vi "Vision Processing.vi"(4 "error in (no error)":errorcluster, 7 "Image Size":T6=enum."320x240") -> ()   [LabVIEW 2015]
doc: "This VI runs in parallel to other tasks. It gets images from the camera, processes them for color or shape and use that information to affect robot behavior."
uses:
  <vilib>/Rock Robotics/WPI/Camera/WPI_CameraImageSize.ctl
  Vision Example/Vision Support Code/Camera Types.ctl
  <vilib>/Rock Robotics/WPI/Camera/WPI_CameraWhite Balance Values.ctl
  <vilib>/Rock Robotics/WPI/Camera/WPI_CameraExposure Values.ctl
  <vilib>/Rock Robotics/WPI/Camera/WPI_CameraFrameRate.ctl
  Robot Global Data.vi
  <vilib>/vision/NI_Vision_Development_Module.lvlib
panel:
  out "ms to process":u32
  in  "LED Color":T1={"Hue"={23.67058792990901, 48.923317529462665}, "Sat"={66.78571428571429, 255.0}, "Val"={48.571428571428584, 255.0}} {"Hue" scale=0.0..255.0 scale format="%#_3g"}
  out "Qualified Particles":i32
  in  "Score Threshold":dbl=75.0
  in  "Aspect Fudge Factor":dbl=1.0
  in  "Min Score Threshold":i32=75
  in  "Camera Type":T2=enum."MS HD3000 square"
  in  "Emphasize Limit Tests":bool=TRUE
  out "Masked":T3(plugin-control)
  in  "Display Mask":bool=TRUE
  out "Original Image":T3(plugin-control)
  in  "Display Original":bool=TRUE
  out "Sorted Particle Scores":T4(array[cluster]) {"Moment Factor" format="%#_3g"; "Aspect Ratio" format="%#_3g"; "Area to CH" format="%#_3g"; "X" format="%#_3g"; "Y" format="%#_3g"}
  out "Highest Avg Score":dbl
  out "Detected Targets":T5(array[cluster]) {"Normalized Rect"."Numeric 5" format="%#_2g"; "Normalized Rect"."Numeric 3" format="%#_2g"; "Normalized Rect"."Numeric 2" format="%#_2g"; "Normalized Rect"."Numeric" format="%#_2g"}
  out "fps":dbl
  # "Density Profile"
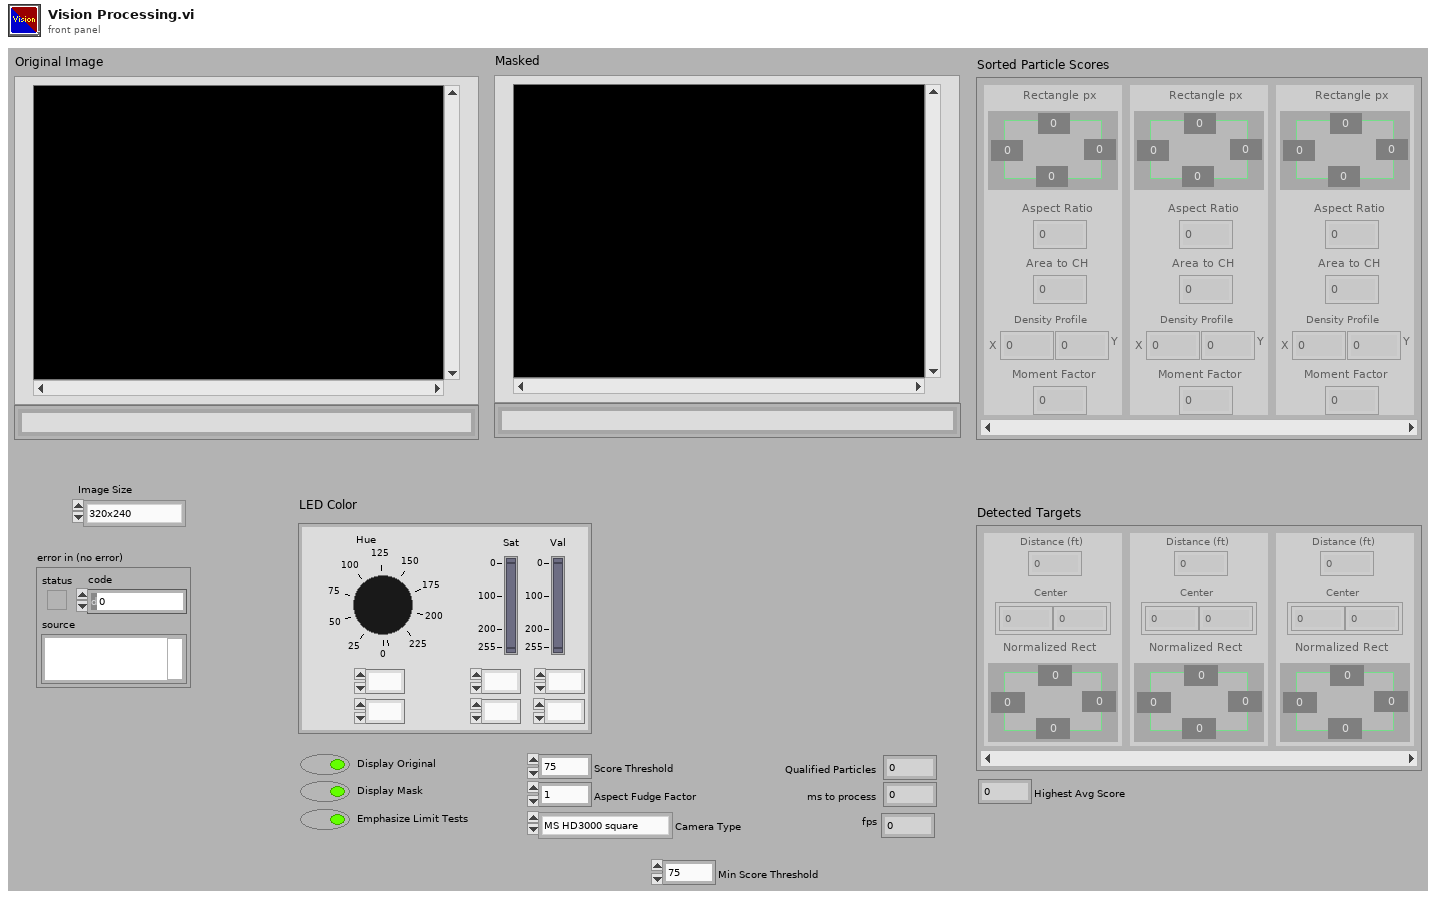
[diagram p1: front panel]
types:
  T1 = cluster{"Hue":cluster{dbl, dbl}, "Sat":cluster{dbl, dbl}, "Val":cluster{dbl, dbl}}
  T2 = typedef "Camera Types.ctl" = enum16{"206", "1011", "1013", "MS HD3000 square", "MS HD3000 640x480"}
  T3 = typedef "IMAQ Image.ctl" = refnum<image>
  T4 = cluster{"Rectangle px":cluster{"Numeric":dbl, "Numeric 2":dbl, "Numeric 3":dbl, "Numeric 5":dbl}, "Aspect Ratio":dbl, "Area to CH":dbl, "X":dbl, "Y":dbl, "Moment Factor":dbl}[]
  T5 = cluster{"Distance (ft)":dbl, "Center":cluster{dbl, dbl}, "Normalized Rect":cluster{"Numeric":dbl, "Numeric 2":dbl, "Numeric 3":dbl, "Numeric 5":dbl}}[]
  T6 = typedef "WPI_CameraImageSize.ctl" = enum16{"640x480", "320x240", "160x120", "Custom"}
  T7 = typedef "WPI_CameraFrameRate.ctl" = u32
  T8 = typedef "WPI_CameraExposure Values.ctl" = enum16{"Auto", "Flicker-free 50 Hz", "Flicker-free 60 Hz", "Hold current", "Custom"}
  T9 = typedef "WPI_CameraWhite Balance Values.ctl" = enum16{"Auto", "Fixed indoor", "Fixed outdoor 1", "Fixed outdoor 2", "Fixed fluorescent 1", "Fixed fluorescent 2", "Hold current", "Custom"}
  T10 = typedef "Particle Parameters" = i32
  T11 = typedef "Image Type" = u32
  T12 = typedef "WPI_CameraDevRef.ctl" = cluster{"Camera Address":string, "CameraStatus":errorcluster}
  T13 = cluster{"Bounding box":cluster{"left":dbl, "top":dbl, "right":dbl, "bottom":dbl}, "Aspect Ratio":dbl, "Area to CH":dbl, "X Mask":dbl, "Y Mask":dbl, "Moment":dbl}[]
  T14 = cluster{"Rectangle":cluster{"Numeric":dbl, "Numeric 2":dbl, "Numeric 3":dbl, "Numeric 5":dbl}, "L":dbl, "Area to CH":dbl, "X":dbl, "Y":dbl, "Moment Factor":dbl}[]
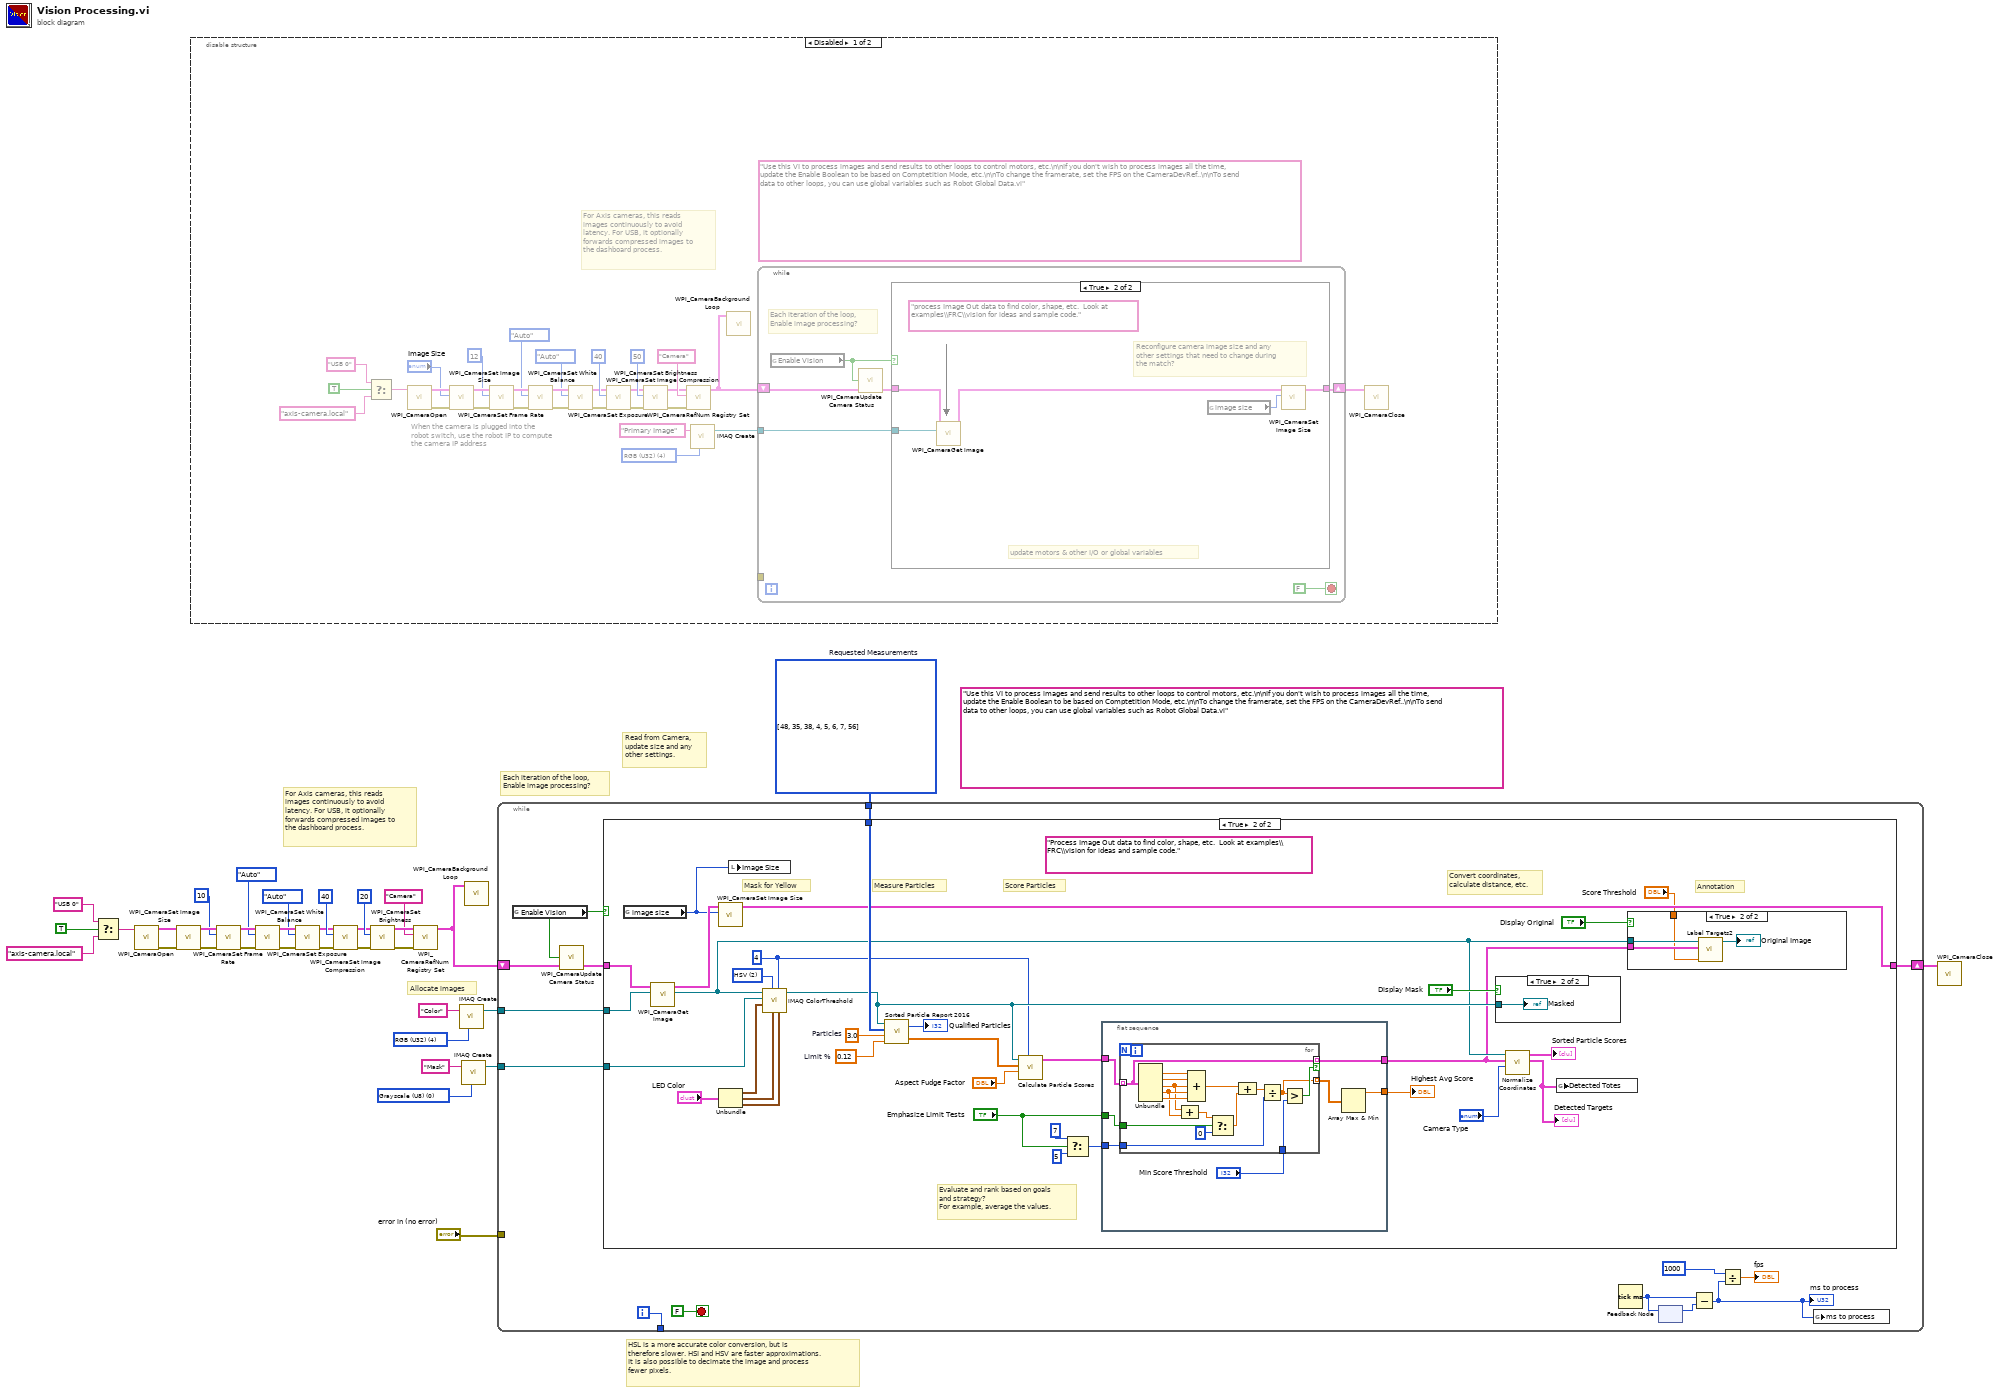
[diagram p0: block diagram]
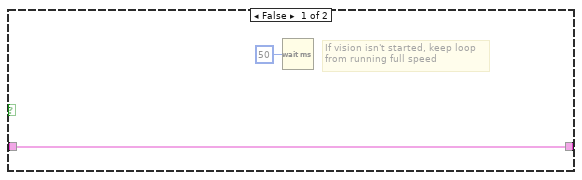
[diagram p2: hidden frame]
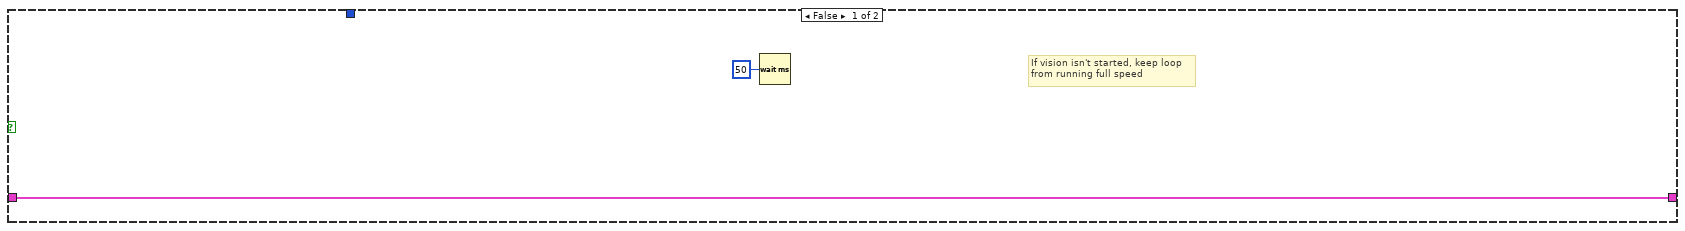
[diagram p4: hidden frame]
diagram:
  (unwired) "Use this VI to process images and send results to other loops to control motors, etc.\n\nIf you don't wish to process images all the time, update the Enable Boolean to be based on Comptetition Mode, etc.\n\nTo change the framerate, set the FPS on the CameraDevRef..\n\nTo send data to other loops, you can use global variables such as Robot Global Data.vi"
  w8 = T10[] [48, 35, 38, 4, 5, 6, 7, 56] items=["Center of Mass X", "Center of Mass Y", "First Pixel X", "First Pixel Y", "Bounding Rect Left", "Bounding Rect Top", "Bounding Rect Right", "Bounding Rect Bottom", "Max Feret Diameter Start X", "Max Feret Diameter Start Y", "Max Feret Diameter End X", "Max Feret Diameter End Y", "Max Horiz. Segment Length Left", "Max Horiz. Segment Length Right", "Max Horiz. Segment Length Row", "-", "Bounding Rect Width", "Bounding Rect Height", "Bounding Rect Diagonal", "Perimeter", "Convex Hull Perimeter", "Holes' Perimeter", "Max Feret Diameter", "Equivalent Ellipse Major Axis", "Equivalent Ellipse Minor Axis", "Equivalent Ellipse Minor Axis (Feret)", "Equivalent Rect Long Side", "Equivalent Rect Short Side", "Equivalent Rect Diagonal", "Equivalent Rect Short Side (Feret)", "Average Horiz. Segment Length", "Average Vert. Segment Length", "Hydraulic Radius", "Waddel Disk Diameter", "-", "Area", "Holes' Area", "Particle & Holes' Area", "Convex Hull Area", "Image Area", "-", "Number of Holes", "Number of Horiz. Segments", "Number of Vert. Segments", "-", "Orientation", "Max Feret Diameter Orientation", "-", "% Area/Image Area", "% Area/(Particle & Holes' Area)", "Ratio of Equivalent Ellipse Axes", "Ratio of Equivalent Rect Sides", "-", "Elongation Factor", "Compactness Factor", "Heywood Circularity Factor", "Type Factor", "-", "Sum X", "Sum Y", "Sum XX", "Sum XY", "Sum YY", "Sum XXX", "Sum XXY", "Sum XYY", "Sum YYY", "-", "Moment of Inertia XX", "Moment of Inertia XY", "Moment of Inertia YY", "Moment of Inertia XXX", "Moment of Inertia XXY", "Moment of Inertia XYY", "Moment of Inertia YYY", "Norm. Moment of Inertia XX", "Norm. Moment of Inertia XY", "Norm. Moment of Inertia YY", "Norm. Moment of Inertia XXX", "Norm. Moment of Inertia XXY", "Norm. Moment of Inertia XYY", "Norm. Moment of Inertia YYY", "Hu Moment 1", "Hu Moment 2", "Hu Moment 3", "Hu Moment 4", "Hu Moment 5", "Hu Moment 6", "Hu Moment 7"]  # Requested Measurements
  w5 = T11 0 items=["Grayscale (U8)", "Grayscale (I16)", "Grayscale (SGL)", "Complex (CSG)", "RGB (U32)", "HSL (U32)", "RGB (U64)", "Grayscale (U16)"] ("Image Type")
  w3 = T11 4 items=["Grayscale (U8)", "Grayscale (I16)", "Grayscale (SGL)", "Complex (CSG)", "RGB (U32)", "HSL (U32)", "RGB (U64)", "Grayscale (U16)"] ("Image Type")
  # "Read from Camera,\nupdate size and any\nother settings."
  # "Each iteration of the loop,\nEnable image processing?"
  # "HSL is a more accurate color conversion, but is\ntherefore slower. HSI and HSV are faster approximations.\nIt is also possible to decimate the image and process\nfewer pixels."
  # "For Axis cameras, this reads\nimages continuously to avoid\nlatency. For USB, it optionally\nforwards compressed images to\nthe dashboard process."
  # "Allocate images"
  n1 = Select(t="USB 0" ("format string"), s=TRUE ("dot notation? (F)"), f="axis-camera.local" ("format string")) -> (s? t:f=w9:string)
  n2 = call <vilib>:"WPI_CameraOpen.vi"("Camera Address"=w9) -> ("error out"=w21:errorcluster, "CameraDevRef"=w22:T12)  [unwired: 2 in, 7 out]
  n3 = call <vilib>:"WPI_CameraSet Image Size.vi"("error in (no error)"=w21, "CameraDevRef"=w22) -> ("error out"=w20:errorcluster, "CameraDevRef Out"=w23:T12)  [unwired: 2 in, 6 out]
  n4 = disable-structure shown="Disabled" {
    frame Disabled {
      (unwired) "Use this VI to process images and send results to other loops to control motors, etc.\n\nIf you don't wish to process images all the time, update the Enable Boolean to be based on Comptetition Mode, etc.\n\nTo change the framerate, set the FPS on the CameraDevRef..\n\nTo send data to other loops, you can use global variables such as Robot Global Data.vi"
      w65 = T11 4 items=["Grayscale (U8)", "Grayscale (I16)", "Grayscale (SGL)", "Complex (CSG)", "RGB (U32)", "HSL (U32)", "RGB (U64)"] ("Image Type")
      # "When the camera is plugged into the\nrobot switch, use the robot IP to compute\nthe camera IP address"
      # "For Axis cameras, this reads\nimages continuously to avoid\nlatency. For USB, it optionally\nforwards compressed images to\nthe dashboard process."
      n5 = Select(t="USB 0" ("format string"), s=TRUE ("dot notation? (F)"), f="axis-camera.local" ("format string")) -> (s? t:f=w36:string)
      n6 = call <vilib>:"WPI_CameraOpen.vi"("Camera Address"=w36) -> ("error out"=w53:errorcluster, "CameraDevRef"=w54:T12)  [unwired: 2 in, 7 out]
      n7 = call <vilib>:"WPI_CameraSet Image Size.vi"("error in (no error)"=w53, "Image Size"="Image Size", "CameraDevRef"=w54) -> ("error out"=w52:errorcluster, "CameraDevRef Out"=w55:T12)  [unwired: 1 in, 6 out]
      n8 = call <vilib>:"WPI_CameraSet Frame Rate.vi"("error in (no error)"=w52, "Frame Rate (fps)"=T7 12, "CameraDevRef"=w55) -> ("error out"=w51:errorcluster, "CameraDevRef Out"=w57:T12)  [unwired: 7 out]
      n9 = call <vilib>:"WPI_CameraSet White Balance.vi"("error in (no error)"=w51, "White Balance"=WPI_CameraWhite_Balance_Values."Auto", "CameraDevRef"=w57) -> ("error out"=w50:errorcluster, "CameraDevRef Out"=w56:T12)  [unwired: 1 in, 6 out]
      n10 = call <vilib>:"WPI_CameraSet Exposure.vi"("error in (no error)"=w50, "Exposure"=WPI_CameraExposure_Values."Auto", "CameraDevRef"=w56) -> ("error out"=w49:errorcluster, "CameraDevRef Out"=w59:T12)  [unwired: 1 in, 6 out]
      n11 = call <vilib>:"WPI_CameraSet Image Compression.vi"("error in (no error)"=w49, "Compression"=40, "CameraDevRef"=w59) -> ("error out"=w48:errorcluster, "CameraDevRef Out"=w58:T12)  [unwired: 7 out]
      n12 = call <vilib>:"WPI_CameraSet Brightness.vi"("error in (no error)"=w48, "Brightness"=50, "CameraDevRef"=w58) -> ("error out"=w46:errorcluster, "CameraDevRef Out"=w47:T12)  [unwired: 7 out]
      n13 = call <vilib>:"WPI_CameraRefNum Registry Set.vi"("error in (no error)"=w46, "refnum name"="Camera", "CameraDevRef"=w47) -> ("CameraDevRef"=w42:T12)  [unwired: 1 in, 7 out]
      n14 = call "IMAQ Create"("Image Name"="Primary Image", "Image Type"=w65) -> ("New Image"=w63:T3)  [unwired: 2 in, 2 out]
      n15 = call <vilib>:"WPI_CameraBackground Loop.vi"("CameraDevRef"=w42) -> ()  [unwired: 11 in]
      n16 = while {
        shift-right: [w70] -> w40
        shift-left: w42 -> [w68]
        tunnel: w63 -> [w69]
        tunnel: [_] -> w39
        stop <- FALSE stop-if-true
        # "Each iteration of the loop,\nEnable image processing?"
        n17 = global read "Robot Global Data.vi" "Enable Vision"() -> (w66:bool)
        n18 = call <vilib>:"WPI_CameraUpdate Camera Status.vi"("CameraDevRef In"=w68, "Enable Vision"=w66) -> ("CameraDevRef Out"=w67:T12)  [unwired: 3 in]
        n19 = case shown="True" w66 {
          tunnel: w69 -> [_ w77]
          tunnel: [w73 w78] -> w70
          tunnel: w67 -> [w73 w75]
          frame False {
            # "If vision isn't started, keep loop\nfrom running full speed"
            n20 = Wait (ms)(milliseconds to wait=u32 50) -> ()  [unwired: 1 out]
          }
          frame True {
            (unwired) "process Image Out data to find color, shape, etc.  Look at examples\\FRC\\vision for ideas and sample code."
            # "update motors & other I/O or global variables"
            # "Reconfigure camera image size and any\nother settings that need to change during\nthe match?"
            n21 = call <vilib>:"WPI_CameraGet Image.vi"("Image"=w77, "CameraDevRef"=w75) -> ("CameraDevRef Out"=w74:T12)  [unwired: 1 in, 8 out]
            n22 = global read "Robot Global Data.vi" "image size"() -> (w76:T6)
            n23 = call <vilib>:"WPI_CameraSet Image Size.vi"("Image Size"=w76, "CameraDevRef"=w74) -> ("CameraDevRef Out"=w78:T12)  [unwired: 2 in, 7 out]
          }
        }
      }
      n24 = call <vilib>:"WPI_CameraClose.vi"("CameraDevRef"=w40) -> ()  [unwired: 1 in, 10 out]
    }
    frame Enabled {
    }
  }
  n25 = call <vilib>:"WPI_CameraSet Frame Rate.vi"("error in (no error)"=w20, "Frame Rate (fps)"=T7 10, "CameraDevRef"=w23) -> ("error out"=w19:errorcluster, "CameraDevRef Out"=w25:T12)  [unwired: 7 out]
  n26 = call <vilib>:"WPI_CameraSet White Balance.vi"("error in (no error)"=w19, "White Balance"=WPI_CameraWhite_Balance_Values."Auto", "CameraDevRef"=w25) -> ("error out"=w18:errorcluster, "CameraDevRef Out"=w24:T12)  [unwired: 1 in, 6 out]
  n27 = call <vilib>:"WPI_CameraSet Exposure.vi"("error in (no error)"=w18, "Exposure"=WPI_CameraExposure_Values."Auto", "CameraDevRef"=w24) -> ("error out"=w17:errorcluster, "CameraDevRef Out"=w27:T12)  [unwired: 1 in, 6 out]
  n28 = call <vilib>:"WPI_CameraSet Image Compression.vi"("error in (no error)"=w17, "Compression"=40, "CameraDevRef"=w27) -> ("error out"=w16:errorcluster, "CameraDevRef Out"=w26:T12)  [unwired: 7 out]
  n29 = call <vilib>:"WPI_CameraSet Brightness.vi"("error in (no error)"=w16, "Brightness"=20, "CameraDevRef"=w26) -> ("error out"=w15:errorcluster, "CameraDevRef Out"=w34:T12)  [unwired: 7 out]
  n30 = call <vilib>:"WPI_CameraRefNum Registry Set.vi"("error in (no error)"=w15, "refnum name"="Camera", "CameraDevRef"=w34) -> ("CameraDevRef"=w31:T12)  [unwired: 1 in, 7 out]
  n31 = call "IMAQ Create"("Image Name"="Color", "Image Type"=w3) -> ("New Image"=w4:T3)  [unwired: 2 in, 2 out]
  n32 = call "IMAQ Create"("Image Name"="Mask", "Image Type"=w5) -> ("New Image"=w7:T3)  [unwired: 2 in, 2 out]
  n33 = call <vilib>:"WPI_CameraBackground Loop.vi"("CameraDevRef"=w31) -> ()  [unwired: 11 in]
  n34 = while {
    tunnel: w4 -> [w87]
    tunnel: w7 -> [w91]
    tunnel: w8 -> [w90]
    tunnel: [w86] -> _
    shift-right: [w82] -> w33
    shift-left: w31 -> [w84]
    tunnel: "error in (no error)" -> [_]
    i -> [w86]
    stop <- FALSE stop-if-true
    n35 = global read "Robot Global Data.vi" "Enable Vision"() -> (w85:bool)
    n36 = call <vilib>:"WPI_CameraUpdate Camera Status.vi"("CameraDevRef In"=w84, "Enable Vision"=w85) -> ("CameraDevRef Out"=w83:T12)  [unwired: 3 in]
    n37 = case shown="True" w85 {
      tunnel: w91 -> [_ w127]
      tunnel: w90 -> [_ w122]
      tunnel: w83 -> [w93 w118]
      tunnel: w87 -> [_ w117]
      tunnel: [w93 w115] -> w82
      frame False {
        # "If vision isn't started, keep loop\nfrom running full speed"
        n38 = Wait (ms)(milliseconds to wait=u32 50) -> ()  [unwired: 1 out]
      }
      frame True {
        w98 = 4 ("Replace Value")
        w112 = u16 2 items=["RGB", "HSL", "HSV", "HSI"] ("Color Mode")
        (unwired) "Process Image Out data to find color, shape, etc.  Look at examples\\FRC\\vision for ideas and sample code."
        w119 = 0.12  # Limit %
        w121 = 3.0  # Particles
        # "Evaluate and rank based on goals\nand strategy?\nFor example, average the values."
        # "Measure Particles"
        # "Convert coordinates,\ncalculate distance, etc."
        # "Annotation"
        # "Score Particles"
        # "Mask for Yellow"
        n39 = global read "Robot Global Data.vi" "image size"() -> (w97:T6)
        n40 = call <vilib>:"WPI_CameraGet Image.vi"("Image"=w117, "CameraDevRef"=w118) -> ("Image Out"=w101:T3, "CameraDevRef Out"=w116:T12)  [unwired: 7 in, 1 out]
        n41 = call <vilib>:"WPI_CameraSet Image Size.vi"("Image Size"=w97, "CameraDevRef"=w116) -> ("CameraDevRef Out"=w115:T12)  [unwired: 2 in, 7 out]
        n42 = Unbundle("LED Color") -> ("Hue"=w126:cluster{dbl, dbl}, "Sat"=w125:cluster{dbl, dbl}, "Val"=w124:cluster{dbl, dbl})
        n43 = local write "Image Size"(w97) -> ()
        n44 = call "IMAQ ColorThreshold"("Blue or Luma or Val or Inten Range"=w124, "Replace Value"=w98, "Green or Sat Range"=w125, "Color Mode"=w112, "Red or Hue Range"=w126, "Image Dst"=w127, "Image Src"=w101) -> ("Image Dst Out"=w111:T3)  [unwired: 3 in, 1 out]
        n45 = call "Sorted Particle Report 2016.vi"("Min Area Size %"=w119, "Particle Count Limit"=w121, "Pixel Measurements"=w122, "Image in"=w111) -> ("Sorted Data"=w110:dbl[][], "Particles"=→"Qualified Particles":i32)
        n46 = call "Calculate Particle Scores.vi"("Pixel Value"=w98, "Aspect Fudge Factor"="Aspect Fudge Factor", "Sorted Data"=w110, "Image in"=w111) -> ("Scores"=w108:T13)  [unwired: 7 in]
        n47 = Select(t=7, s="Emphasize Limit Tests", f=5) -> (s? t:f=w105:i32)
        n48 = flat-sequence {
          tunnel: w108 -> [w138]
          tunnel: w105 -> [w136]
          tunnel: [w139] -> w104
          tunnel: [w133] -> w100
          tunnel: "Emphasize Limit Tests" -> [w137]
          frame #0 {
            n49 = for {
              tunnel: w138 -> [w153] mode=indexing
              tunnel: [w153] -> w133 mode=indexing if=w152
              tunnel: [w151] -> w134 mode=indexing
              tunnel: w136 -> [w150]
              tunnel: "Min Score Threshold" -> [w149]
              tunnel: w137 -> [w142]
              n50 = Unbundle(w153) -> ("Aspect Ratio"=w155:dbl, "Area to CH"=w154:dbl, "X Mask"=w144:dbl, "Y Mask"=w145:dbl, "Moment"=w146:dbl)  [unwired: 1 out]
              n51 = Compound Arithmetic op=ADD(w144, w145) -> (w143:dbl)
              n52 = Compound Arithmetic op=ADD(w155, w154, w144, w145, w146) -> (w148:dbl)
              n53 = Select(t=w143, s=w142, f=0) -> (s? t:f=w141:dbl)
              n54 = Compound Arithmetic op=ADD(w148, w141) -> (w147:dbl)
              n55 = Divide(x=w147, y=w150) -> (x/y=w151:dbl)
              n56 = Greater?(x=w151, y=w149) -> (0:w152:bool)
            }
            n57 = Array Max & Min(array=w134) -> (max value=w139:dbl)  [unwired: 3 out]
          }
        }
        n58 = case shown="True" "Display Mask" {
          tunnel: w111 -> [_ w132]
          frame False {
          }
          frame True {
            "Masked" <- w132
          }
        }
        n59 = call "Normalize Coordinates.vi"("Camera Type"="Camera Type", "Targets"=w100, "Image in"=w101) -> ("Found Targets"=w95:T5, "Sorted Scores"=→"Sorted Particle Scores":T14)  [unwired: 7 in]
        "Detected Targets" <- w95
        n60 = global write "Robot Global Data.vi" "Detected Totes"(w95) -> ()
        n61 = case shown="True" "Display Original" {
          tunnel: w101 -> [_ w131]
          tunnel: w100 -> [_ w129]
          tunnel: "Score Threshold" -> [_ w128]
          frame False {
          }
          frame True {
            n62 = call "Label Targets2.vi"("Score Threshold"=w128, "Targets"=w129, "Image in"=w131) -> ("Image out"=→"Original Image":T3)  [unwired: 8 in]
          }
        }
        "Highest Avg Score" <- w104
      }
    }
    n63 = Tick Count (ms)() -> (millisecond timer value=w88:u32)
    n64 = feedback-in #1(w88) -> ()
    n65 = feedback #1() -> (w89:u32)  [unwired: 1 in]
    n66 = Subtract(x=w88, y=w89) -> (x-y=w81:u32)
    "ms to process" <- w81
    n67 = Divide(x=1000 ("Brightness"), y=w81) -> (x/y=→"fps":dbl)
    n68 = global write "Robot Global Data.vi" "ms to process"(w81) -> ()
  }
  n69 = call <vilib>:"WPI_CameraClose.vi"("CameraDevRef"=w33) -> ()  [unwired: 1 in, 10 out]
